vi "Save System Configuration.vi"(8 "error in (no error)":errorcluster, 10 "System Configuration File Path":path, 11 "System Configuration":T1) -> (0 "error out":errorcluster)   [LabVIEW 2024]
doc: "Saves the system configuration to the configuration file."
uses:
  Controls/Server/System Configuration.ctl
  Controls/Server/Subsystem Configuration.ctl
  <vilib>/Utility/config.llb/Write Key (String).vi
  <vilib>/Utility/config.llb/Write Key (Boolean).vi
  <vilib>/Utility/config.llb/Write Key (U32).vi
  <vilib>/Utility/config.llb/NI_LVConfig.lvlib
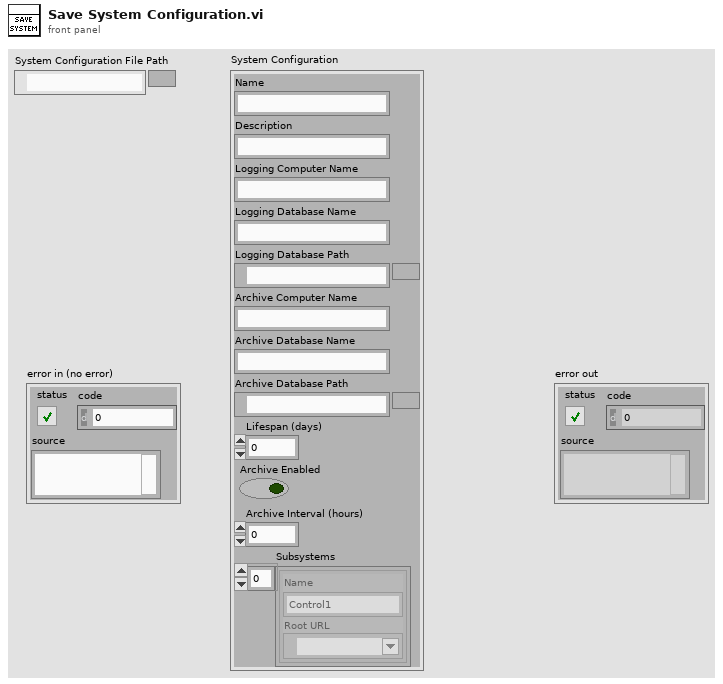
[diagram p1: front panel]
types:
  T1 = typedef "System Configuration.ctl" = cluster{"Name":string, "Description":string, "Logging Computer Name":string, "Logging Database Name":string, "Logging Database Path":path, "Archive Computer Name":string, "Archive Database Name":string, "Archive Database Path":path, "Lifespan (days)":u32, "Archive Enabled":bool, "Archive Interval (hours)":u32, "Subsystems":T2[]}
  T2 = typedef "Subsystem Configuration.ctl" = cluster{"Name":string, "Root URL":refnum<k21>}
  T3 = typedef "NI_LVConfig.lvlib/Config Data RefNum.ctl" = refnum<k1>
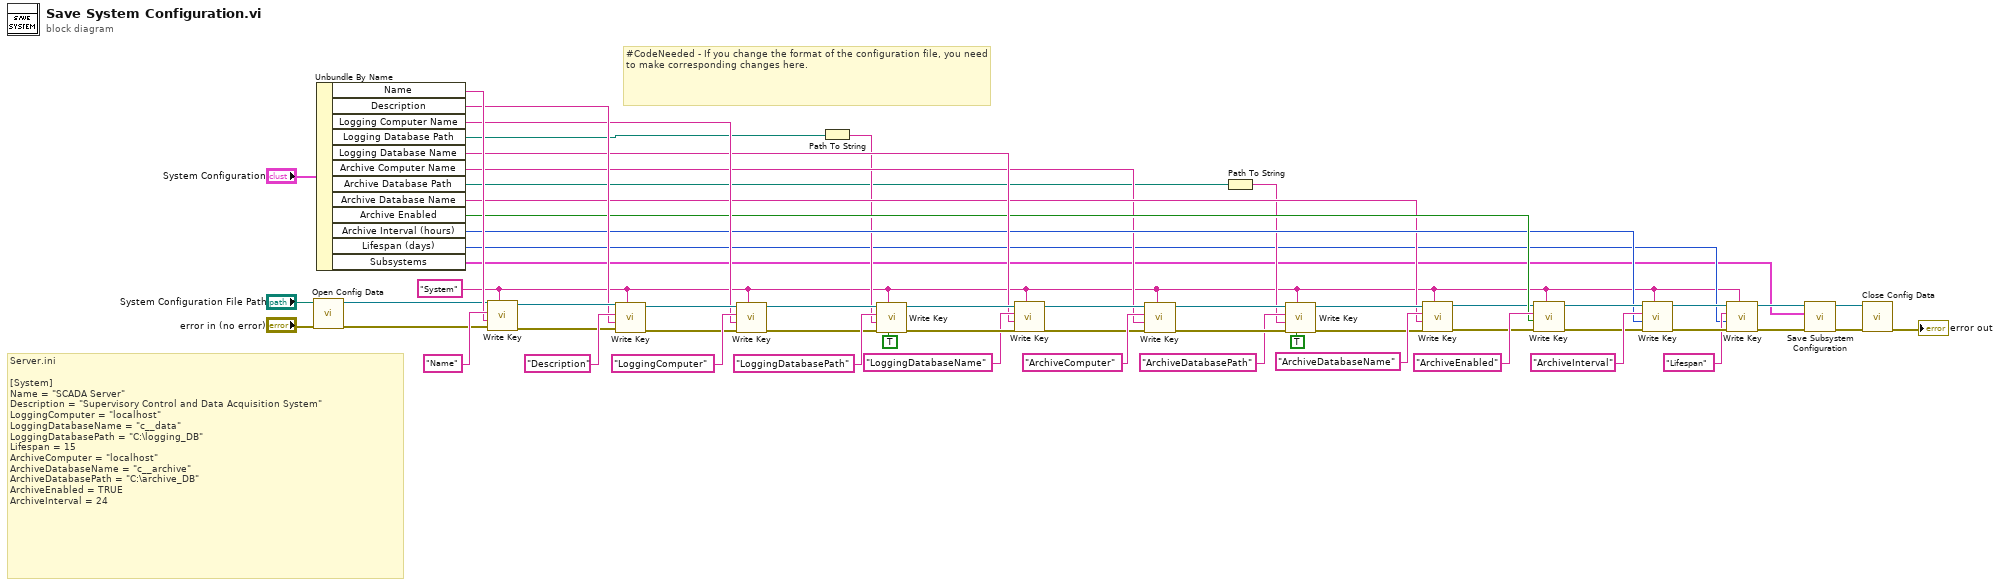
[diagram p0: block diagram]
diagram:
  w10 = "System" ("section")
  # "#CodeNeeded - If you change the format of the configuration file, you need to make corresponding changes here."
  # "Server.ini\n\n[System]\nName = \"SCADA Server\"\nDescription = \"Supervisory Control and Data Acquisition System\"\nLoggingComputer = \"localhost\"\nLoggingDatabaseName = \"c__data\"\nLoggingDatabasePath = \"C:\\logging_DB\"\nLifespan = 15    \nArchiveComputer = \"localhost\"\nArchiveDatabaseName = \"c__archive\"\nArchiveDatabasePath = \"C:\\archive_DB\"\nArchiveEnabled = TRUE    \nArchiveInterval = 24"
  n1 = call <vilib>:"Open Config Data.vi"("error in (no error)"="error in (no error)", "configuration file path"="System Configuration File Path") -> ("error out"=w8:errorcluster, "refnum"=w9:T3)  [unwired: 7 in, 1 out]
  n2 = Unbundle By Name("System Configuration") -> ("Name"=w37:string, "Description"=w36:string, "Logging Computer Name"=w35:string, "Logging Database Path"=w17:path, "Logging Database Name"=w34:string, "Archive Computer Name"=w19:string, "Archive Database Path"=w15:path, "Archive Database Name"=w20:string, "Archive Enabled"=w33:bool, "Archive Interval (hours)"=w32:u32, "Lifespan (days)"=w11:u32, "Subsystems"=w4:T2[])
  n3 = call-poly <vilib>:"Write Key.vi"("section"=w10, "error in (no error)"=w8, "value"=w37, "key"="Name", "refnum"=w9) -> ("error out"=w51:errorcluster, "refnum out"=w52:T3)  [unwired: 4 in, 1 out]
  n4 = call-poly <vilib>:"Write Key.vi"("section"=w10, "error in (no error)"=w51, "value"=w36, "key"="Description", "refnum"=w52) -> ("error out"=w48:errorcluster, "refnum out"=w49:T3)  [unwired: 4 in, 1 out]
  n5 = call-poly <vilib>:"Write Key.vi"("section"=w10, "error in (no error)"=w48, "value"=w35, "key"="LoggingComputer", "refnum"=w49) -> ("error out"=w45:errorcluster, "refnum out"=w46:T3)  [unwired: 4 in, 1 out]
  n6 = Path To String(path=w17) -> (string=w18:string)
  n7 = call-poly <vilib>:"Write Key.vi"("write raw string? (F)"=TRUE, "section"=w10, "error in (no error)"=w45, "value"=w18, "key"="LoggingDatabasePath", "refnum"=w46) -> ("error out"=w44:errorcluster, "refnum out"=w42:T3)  [unwired: 3 in, 1 out]
  n8 = call-poly <vilib>:"Write Key.vi"("section"=w10, "error in (no error)"=w44, "value"=w34, "key"="LoggingDatabaseName", "refnum"=w42) -> ("error out"=w23:errorcluster, "refnum out"=w24:T3)  [unwired: 4 in, 1 out]
  n9 = call-poly <vilib>:"Write Key.vi"("section"=w10, "error in (no error)"=w23, "value"=w19, "key"="ArchiveComputer", "refnum"=w24) -> ("error out"=w28:errorcluster, "refnum out"=w27:T3)  [unwired: 4 in, 1 out]
  n10 = Path To String(path=w15) -> (string=w16:string)
  n11 = call-poly <vilib>:"Write Key.vi"("write raw string? (F)"=TRUE, "section"=w10, "error in (no error)"=w28, "value"=w16, "key"="ArchiveDatabasePath", "refnum"=w27) -> ("error out"=w29:errorcluster, "refnum out"=w31:T3)  [unwired: 3 in, 1 out]
  n12 = call-poly <vilib>:"Write Key.vi"("section"=w10, "error in (no error)"=w29, "value"=w20, "key"="ArchiveDatabaseName", "refnum"=w31) -> ("error out"=w21:errorcluster, "refnum out"=w22:T3)  [unwired: 4 in, 1 out]
  n13 = call-poly <vilib>:"Write Key.vi"("section"=w10, "error in (no error)"=w21, "value"=w33, "key"="ArchiveEnabled", "refnum"=w22) -> ("error out"=w38:errorcluster, "refnum out"=w39:T3)  [unwired: 4 in, 1 out]
  n14 = call-poly <vilib>:"Write Key.vi"("section"=w10, "error in (no error)"=w38, "value"=w32, "key"="ArchiveInterval", "refnum"=w39) -> ("error out"=w13:errorcluster, "refnum out"=w14:T3)  [unwired: 4 in, 1 out]
  n15 = call-poly <vilib>:"Write Key.vi"("section"=w10, "error in (no error)"=w13, "value"=w11, "key"="Lifespan", "refnum"=w14) -> ("error out"=w7:errorcluster, "refnum out"=w6:T3)  [unwired: 4 in, 1 out]
  n16 = call "Save Subsystem Configuration.vi"("error in (no error)"=w7, "Subsystems"=w4, "Configuration Refnum In"=w6) -> ("error out"=w56:errorcluster, "Configuration Refnum Out"=w57:T3)  [unwired: 7 in]
  n17 = call <vilib>:"Close Config Data.vi"("error in (no error)"=w56, "refnum"=w57) -> ("error out"=→"error out":errorcluster)  [unwired: 8 in, 1 out]
